vi "AlliGator Calibration Phasor String.vi"(8 "Error In":errorcluster, 11 "Calibration Phasor":T1) -> (0 "Error Out":errorcluster, 3 "Message":string)   [LabVIEW 2021, in "AlliGator Phasor Calibration.lvlib"]
doc: "Builds calibration phasor string."
uses:
  Phasor/Calibration Phasor (m, phi).ctl
  AlliGator Phasor Calibration.lvlib
  Phasor/Phasor.lvlib
panel:
  # "see the AlliGator License on the block diagram (Ctrl+E or Window:Show Block Diagram)"
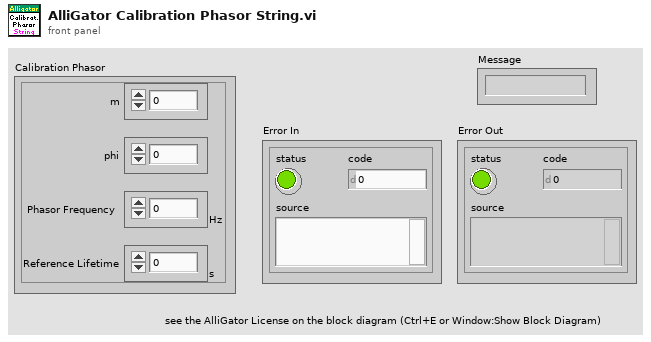
[diagram p1: front panel]
types:
  T1 = typedef "Phasor.lvlib/Calibration Phasor (m, phi).ctl" = cluster{"m":dbl, "phi":dbl, "Phasor Frequency":dbl[unit], "Reference Lifetime":dbl[unit]}
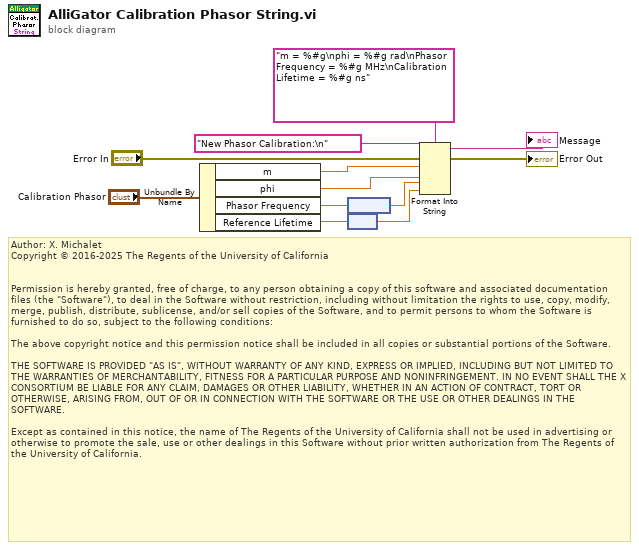
[diagram p0: block diagram]
diagram:
  # "Author: X. Michalet\nCopyright © 2016-2025 The Regents of the University of California\n \n\nPermission is hereby granted, free of charge, to any person obtaining a copy of this software and associated documentation files (the \"Software\"), to deal in the Software without restriction, including without limitation the rights to use, copy, modify, merge, publish, distribute, sublicense, and/or sell copies of the Software, and to permit persons to whom the Software is furnished to do so, subject to the following conditions:\n\nThe above copyright notice and this permission notice shall be included in all copies or substantial portions of the Software.\n\nTHE SOFTWARE IS PROVIDED \"AS IS\", WITHOUT WARRANTY OF ANY KIND, EXPRESS OR IMPLIED, INCLUDING BUT NOT LIMITED TO THE WARRANTIES OF MERCHANTABILITY, FITNESS FOR A PARTICULAR PURPOSE AND NONINFRINGEMENT. IN NO EVENT SHALL THE X CONSORTIUM BE LIABLE FOR ANY CLAIM, DAMAGES OR OTHER LIABILITY, WHETHER IN AN ACTION OF CONTRACT, TORT OR OTHERWISE, ARISING FROM, OUT OF OR IN CONNECTION WITH THE SOFTWARE OR THE USE OR OTHER DEALINGS IN THE SOFTWARE.\n\nExcept as contained in this notice, the name of The Regents of the University of California shall not be used in advertising or otherwise to promote the sale, use or other dealings in this Software without prior written authorization from The Regents of the University of California."
  n1 = Unbundle By Name("Calibration Phasor") -> ("m"=w11:dbl, "phi"=w9:dbl, "Phasor Frequency"=w6:dbl[unit], "Reference Lifetime"=w4:dbl[unit])
  n2 = node(w6) -> (w5:dbl)
  n3 = node(w4) -> (w3:dbl)
  n4 = Format Into String(format string="m = %#g\nphi = %#g rad\nPhasor Frequency = %#g MHz\nCalibration Lifetime = %#g ns" ("Label"), initial string="New Phasor Calibration:\n", error in="Error In", w11, w9, w5, w3) -> (resulting string=→"Message":string, error out=→"Error Out":errorcluster)
